vi "read single tc.vi"(8 "error in (no error)":errorcluster, 10 "Index":u32, 11 "hardware in":refnum<class "hardware.lvclass">) -> (0 "error out":errorcluster, 2 "Temp":dbl, 3 "hardware out":refnum<class "hardware.lvclass">)   [LabVIEW 2025, in "hardware.lvclass"]
uses:
  hardware.lvclass
  hardware.lvclass/hardware.ctl
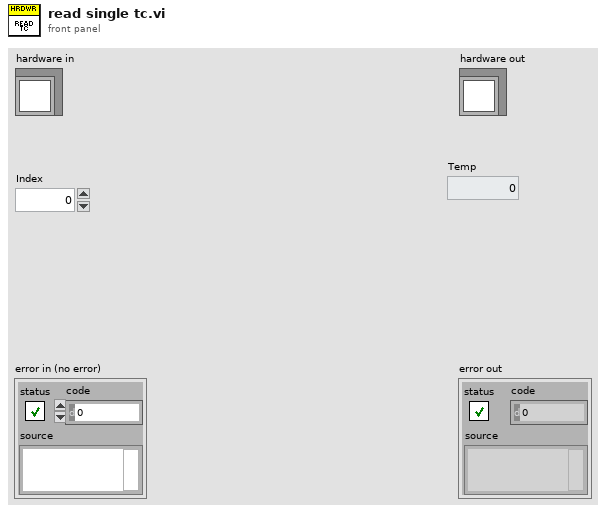
[diagram p1: front panel]
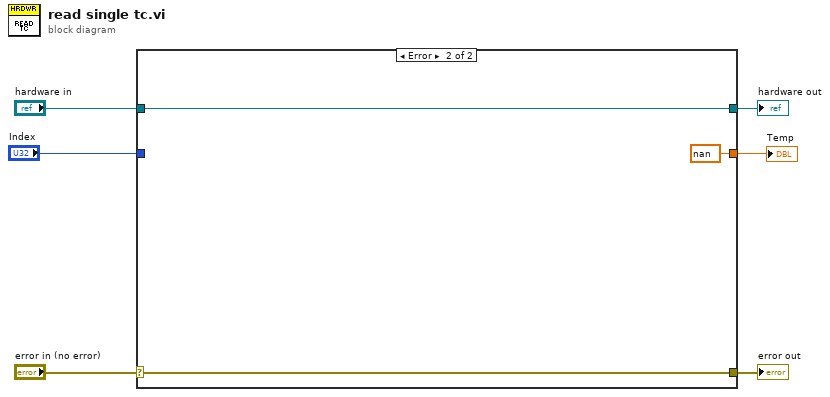
[diagram p0: block diagram]
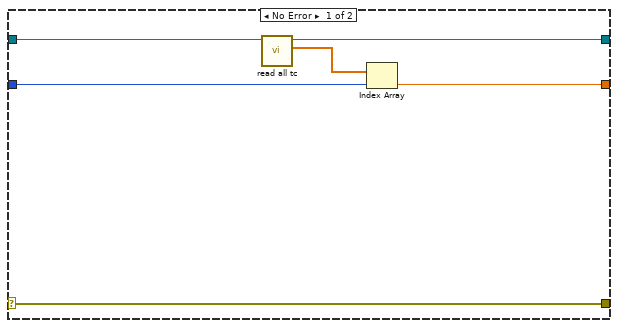
[diagram p2: hidden frame]
diagram:
  n1 = case shown="Error" "error in (no error)" {
    selector: "error in (no error)" -> [w12 w15]
    tunnel: [w12 w15] -> w5
    tunnel: [w10 w14] -> w3
    tunnel: "hardware in" -> [w11 w14]
    tunnel: "Index" -> [w8 _]
    tunnel: [w7 nan ("Waveform")] -> w1
    frame No Error {
      n2 = call-dynamic "read all tc.vi"("hardware in"=w11) -> ("data"=w9:dbl[], "hardware out"=w10:refnum<class "hardware.lvclass">)  [unwired: 8 in, 1 out]
      n3 = Index Array(array=w9, index=w8) -> (element=w7:dbl)
    }
    frame Error {
    }
  }
  "error out" <- w5
  "hardware out" <- w3
  "Temp" <- w1
